vi "Current VI Path.vi"(1 "Time":i32) -> (0 "VI path":path)   [LabVIEW 2018]
panel:
  out "Application Directory":path
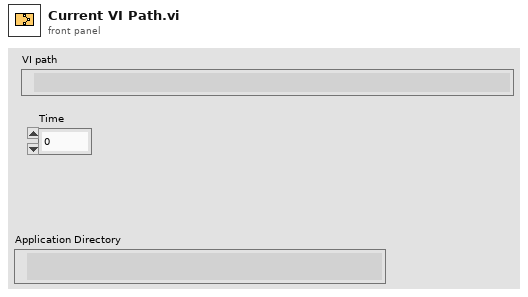
[diagram p1: front panel]
types:
  T1 = enum32{"invalid app kind", "Development System", "Run Time System", "Student Edition", "Embedded LabVIEW", "Evaluation", "Custom"}
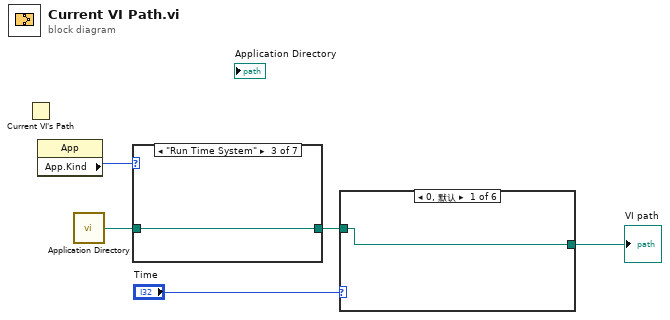
[diagram p0: block diagram]
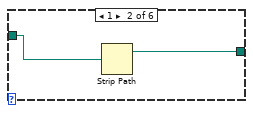
[diagram p8: hidden frame]
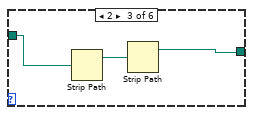
[diagram p9: hidden frame]
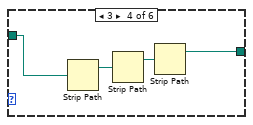
[diagram p10: hidden frame]
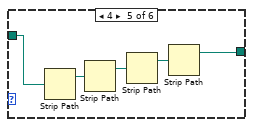
[diagram p11: hidden frame]
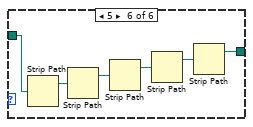
[diagram p12: hidden frame]
diagram:
  n1 = Current VI's Path() -> ()  [unwired: 1 out]
  n2 = property class="App"() -> ("App.Kind"=w3:T1)  [unwired: 2 in, 2 out]
  n3 = call <vilib>:"Application Directory.vi"() -> ("Application Directory"=w1:path)
  n4 = case shown="\"Run Time System\"" w3 {
    tunnel: w1 -> [w6 w7 w8 w9 w10 w11 w12]
    tunnel: [w6 w7 w8 w9 w10 w11 w12] -> w2
    frame "invalid app kind", Default {
    }
    frame "Development System" {
    }
    frame "Run Time System" {
    }
    frame "Student Edition" {
    }
    frame "Embedded LabVIEW" {
    }
    frame "Evaluation" {
    }
    frame "Custom" {
    }
  }
  n5 = case shown="0, 默认" "Time" {
    tunnel: w2 -> [w13 w15 w16 w19 w23 w28]
    tunnel: [w13 w14 w17 w20 w24 w29] -> w4
    frame 0, Default {
    }
    frame 1 {
      n6 = Strip Path(path=w15) -> (stripped path=w14:path)  [unwired: 1 out]
    }
    frame 2 {
      n7 = Strip Path(path=w16) -> (stripped path=w18:path)  [unwired: 1 out]
      n8 = Strip Path(path=w18) -> (stripped path=w17:path)  [unwired: 1 out]
    }
    frame 3 {
      n9 = Strip Path(path=w19) -> (stripped path=w22:path)  [unwired: 1 out]
      n10 = Strip Path(path=w22) -> (stripped path=w21:path)  [unwired: 1 out]
      n11 = Strip Path(path=w21) -> (stripped path=w20:path)  [unwired: 1 out]
    }
    frame 4 {
      n12 = Strip Path(path=w23) -> (stripped path=w27:path)  [unwired: 1 out]
      n13 = Strip Path(path=w27) -> (stripped path=w25:path)  [unwired: 1 out]
      n14 = Strip Path(path=w25) -> (stripped path=w26:path)  [unwired: 1 out]
      n15 = Strip Path(path=w26) -> (stripped path=w24:path)  [unwired: 1 out]
    }
    frame 5 {
      n16 = Strip Path(path=w28) -> (stripped path=w33:path)  [unwired: 1 out]
      n17 = Strip Path(path=w33) -> (stripped path=w31:path)  [unwired: 1 out]
      n18 = Strip Path(path=w31) -> (stripped path=w32:path)  [unwired: 1 out]
      n19 = Strip Path(path=w32) -> (stripped path=w30:path)  [unwired: 1 out]
      n20 = Strip Path(path=w30) -> (stripped path=w29:path)  [unwired: 1 out]
    }
  }
  "VI path" <- w4
